vi "NACA_0015_Pressure_with_profile.vi"(3 "Mode":T5, 5 "Traverse line In":T1 {"Row Duration (mins)" format="%#.1f"; "Row No" min=0; "Trace Gas Concentration (%)" min=0.0 format="%#.2f"; "Emission Rate (l/min)" format="%#.2f"; "Tunnel Speed" format="%#.2f"; "Start X" format="%#.2f"; "Start Y" format="%#.2f"; "Start Z" format="%#.2f"; "End X" format="%#.2f"; "End Y" format="%#.2f"; "End Z" format="%#.2f"; "Averaging time (min)" min=0.0 format="%#.2f"}) -> (0 "Error Message":string, 1 "Status":T4, 2 "Traverse line Out":T1 {"Row Duration (mins)" format="%#.1f"; "Row No" min=0; "Trace Gas Concentration (%)" min=0.0 format="%#.2f"; "Emission Rate (l/min)" format="%#.2f"; "Tunnel Speed" format="%#.2f"; "Start X" format="%#.2f"; "Start Y" format="%#.2f"; "Start Z" format="%#.2f"; "End X" format="%#.2f"; "End Y" format="%#.2f"; "End Z" format="%#.2f"; "Averaging time (min)" min=0.0 format="%#.2f"})   [LabVIEW 2011]
uses:
  Gen Trav/Traverse_cluster.ctl
  Gen Trav/Spacing.ctl
  Controls/Multi_run_mode.ctl
  Controls/User_Specific_mode.ctl
  Gen Trav/Multi_Run_Status.ctl
  Gen Trav/Trav_mode.ctl
  Controls/Save_Data.ctl
  Controls/Setup.ctl
  <vilib>/Analysis/1siggen.llb/Ramp Pattern by Delta.vi
  <vilib>/Analysis/1siggen.llb/Ramp Pattern by Samples.vi
  Globals/Extra_Commands_Global.vi
  Globals/Meas_global.vi
  <vilib>/Analysis/NI_AALBase.lvlib
panel:
  out "Profile Points":cluster{dbl[], dbl[]}[](graph)
  out "Wake Profile":cluster{dbl[], dbl[]}(graph)
  in  "stop":bool
  out "Pressure":cluster{dbl[], dbl[]}(graph)
  out "Measurement No":i32
  # "X           Y            Z"
  # "Start"
  # "End"
  # "X           Y            Z"
  # "Start"
  # "End"
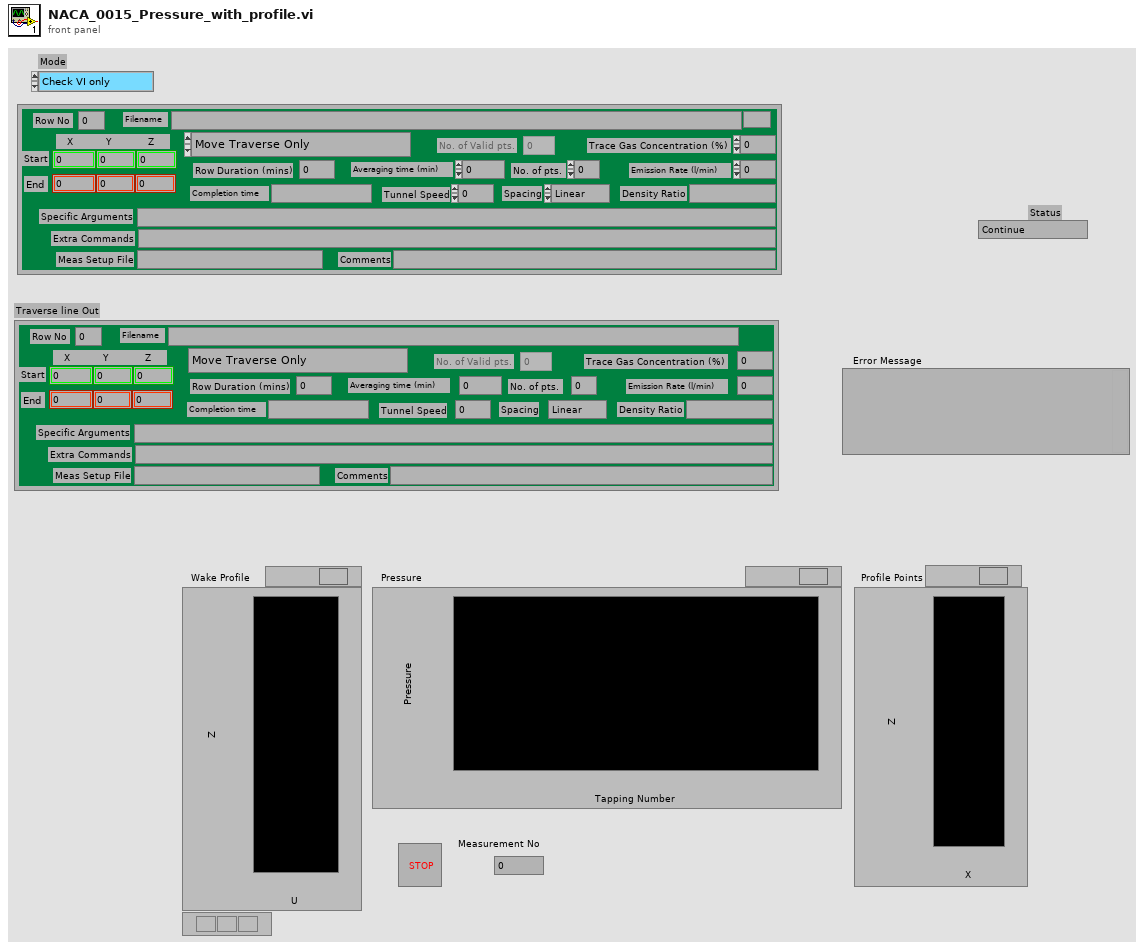
[diagram p1: front panel]
types:
  T1 = typedef "Traverse_cluster.ctl" = cluster{"Start X":dbl, "Start Y":dbl, "Start Z":dbl, "End X":dbl, "End Y":dbl, "End Z":dbl, "No. of pts.":i32, "Spacing":T2, "Filename":path, "Tunnel Speed":dbl, "Averaging time (min)":dbl, "Extra Commands":string, "Specific Arguments":string, "Emission Rate (l/min)":dbl, "Trace Gas Concentration (%)":dbl, "Density Ratio":string, "Comments":string, "Row No":i32, "Row Type Selector":T3, "Completion time":string, "Row Duration (mins)":dbl, "No. of Valid pts.":i32, "Meas Setup File":string}
  T2 = typedef "Spacing.ctl" = enum16{"Linear", "Log", "Gauss", "Specified", "N/A"}
  T3 = typedef "Multi_run_mode.ctl" = enum16{"Move Traverse Only", "Set Tunnel Speed Only", "Set Source Only", "Set Measurement Conditions", "Single Measurement", "Vertical Profile", "Lateral Profile", "Longitudinal Profile", "Explore Volume", "Multi-Axis Profile", "Auto Calibrate", "Meas Fast FID Bkgnd", "Check Beam Power", "Scanning Valve Measurement", "Run VI Named:", "Set ADAM Ch", "Wait (minutes)", "Send Message", "Synchronize With:", "Fall Back to this Row", "Turn Off Row Repeating", "Blank Row", "Traverse 3D Volume"}
  T4 = typedef "Multi_Run_Status.ctl" = enum16{"Continue", "Jump to Next Point", "Jump to Next Row", "Jump To Fall Back", "Terminate Run"}
  T5 = typedef "User_Specific_mode.ctl" = enum16{"Check VI only", "Run VI"}
  T6 = typedef "Trav_mode.ctl" = enum16{"Move traverse", "Read traverse position", "Teach Position"}
  T7 = typedef "Save_Data.ctl" = enum16{"Save No Data", "Save Data"}
  T8 = typedef "Setup.ctl" = enum16{"Run Program", "Show Setup", "Save Current Setup", "Setup Front Panel"}
  T9 = typedef "Status_Cluster.ctl" = cluster{"Status":T4, "Error Type":string, "Error Description":string}
  T10 = typedef "Analysis_info_cluster.ctl" = cluster{"Colour":u32, "Inst type":T11, "Inst name":string, "Symbol":string, "Code name":string, "Extra Info":string, "Inst Array":T12, "Extra Titles":string[], "Extra Values":string[], "U":dbl, "u^2":dbl, "u^3":dbl, "u^4":dbl, "Skew_u":dbl, "Kurt_u":dbl, "Sd Error in Mean":dbl, "% u'/U":dbl, "X":dbl, "Y":dbl, "Z":dbl, "Timescale integral to 25%":dbl, "Sd Error in Variance":dbl, "Calib File":path, "Calib Constants":dbl[], "Output Position":bool, "Full Stats":bool, "Av Sampling Rate":dbl, "Av No of Samples":dbl, "Total Meas Time (s)":dbl, "ADAM Ch Name":string}
  T11 = typedef "Inst_type.ctl" = enum16{"Propeller anemometer", "Raw voltage", "Pressure Transducer", "Pitot-static tube", "Preston tube", "Hot wire", "Cross wire 1", "Cross wire 2", "Generic Linear", "Generic Polynomial", "Generic BackPoly", "Fast FID", "Thermocouple", "Cold wire", "Pulsed Wire", "LDA Vel", "LDA Tran time", "LDA Arr time"}
  T12 = typedef "Instrument_Array.ctl" = enum16{"PWA", "LDA", "Analogue"}
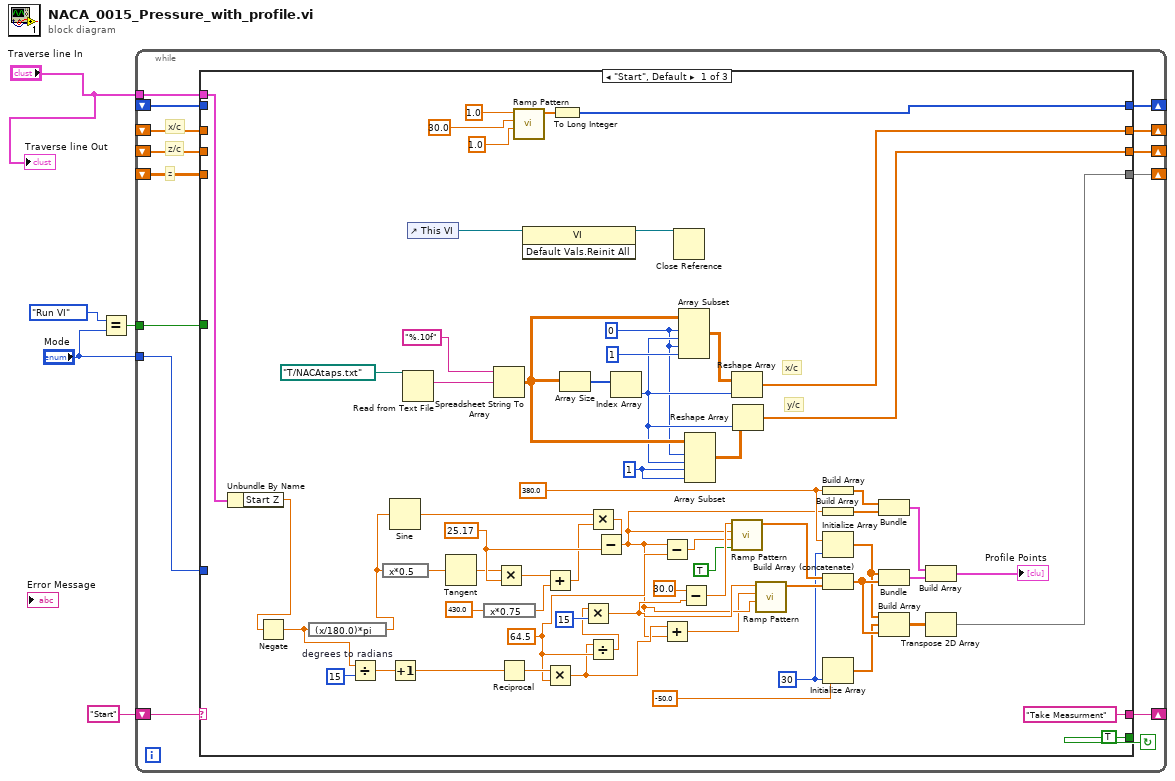
[diagram p0: block diagram]
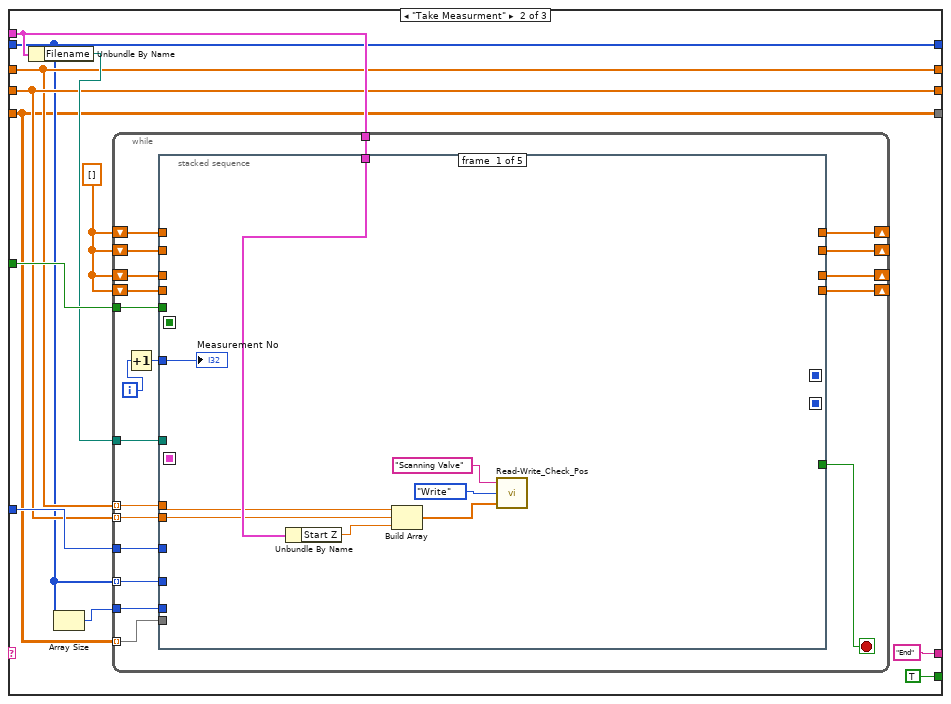
[diagram p2: hidden frame]
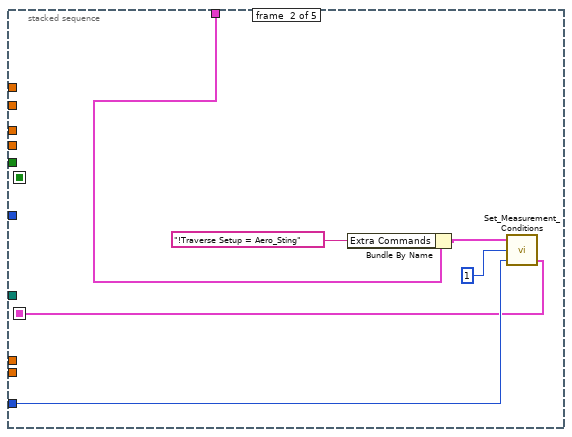
[diagram p3: hidden frame]
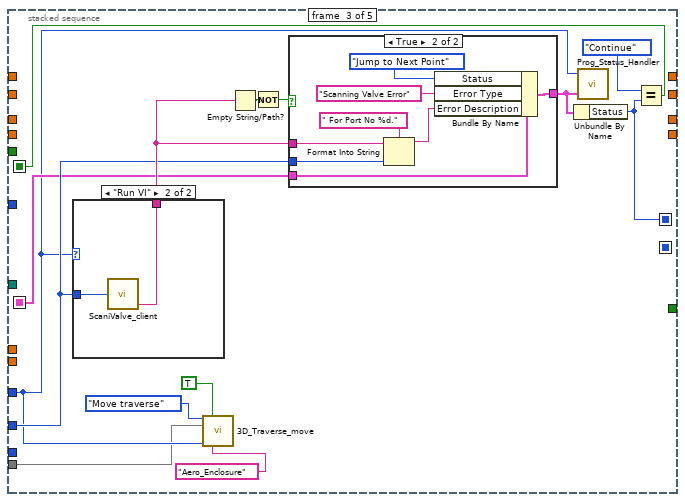
[diagram p4: hidden frame]
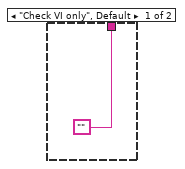
[diagram p5: hidden frame]
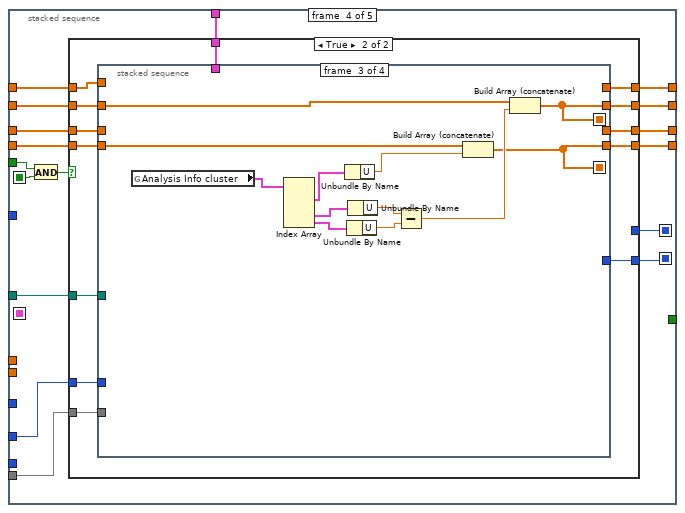
[diagram p7: hidden frame]
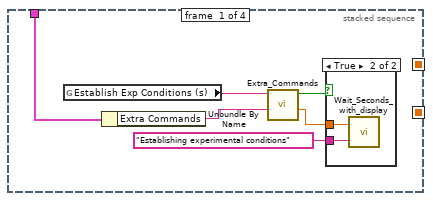
[diagram p9: hidden frame]
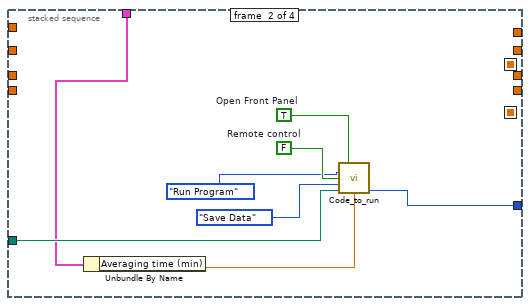
[diagram p11: hidden frame]
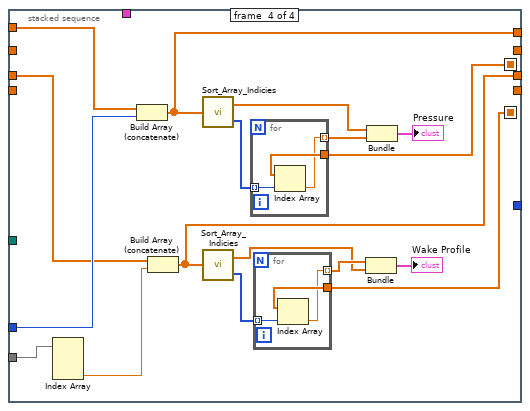
[diagram p12: hidden frame]
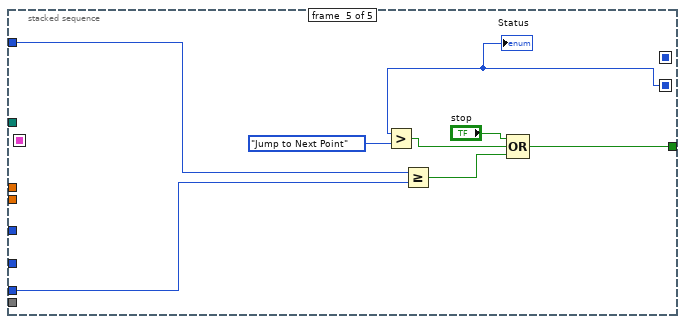
[diagram p13: hidden frame]
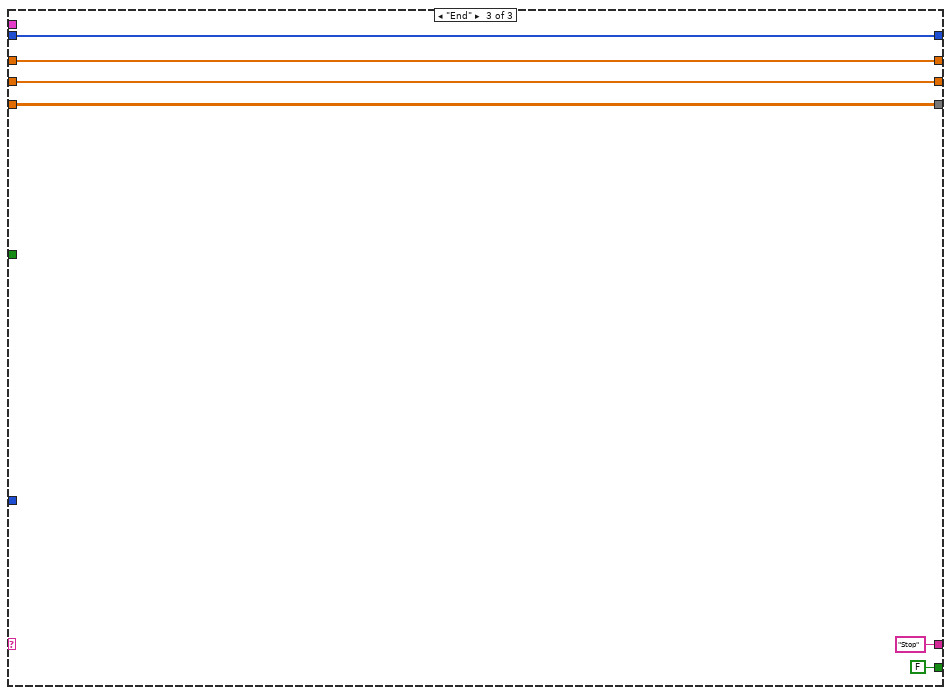
[diagram p14: hidden frame]
diagram:
  n1 = Equal?(x=User_Specific_mode."Run VI" ("Mode"), y="Mode") -> (x = y?=w2:bool)
  n2 = while {
    tunnel: "Traverse line In" -> [w18]
    shift-right: [w17] -> _
    shift-left: "Start" -> [w16]
    tunnel: "Mode" -> [w15]
    tunnel: w2 -> [w14]
    shift-right: [w13] -> _
    shift-left: _ -> [w12]
    shift-right: [w11] -> _
    shift-left: _ -> [w9]
    shift-right: [w10] -> _
    shift-left: _ -> [w8]
    shift-right: [w7] -> _
    shift-left: _ -> [w6]
    stop <- w19 continue-if-true
    # "z"
    # "z/c"
    # "x/c"
    n3 = case shown="\"Start\", Default" w16 {
      tunnel: [TRUE TRUE FALSE] -> w19
      tunnel: w18 -> [w62 w93 _]
      tunnel: ["Take Measurment" "End" "Stop"] -> w17
      tunnel: w15 -> [_ w91 _]
      tunnel: w14 -> [_ w94 _]
      tunnel: [w80 w88 w254] -> w13
      tunnel: w12 -> [_ w88 w254]
      tunnel: [w66 w89 w253] -> w11
      tunnel: [w65 w90 w252] -> w10
      tunnel: w9 -> [_ w89 w253]
      tunnel: w8 -> [_ w90 w252]
      tunnel: [w22 w86 w251] -> w7
      tunnel: w6 -> [_ w86 w251]
      frame "Start", Default {
        w46 = 380.0 ("X")
        w52 = 64.5 ("y")
        w33 = 25.17 ("y")
        w23 = 30 ("dimension size")
        w67 = 1 ("index")
        w68 = 0 ("index")
        # "y/c"
        # "x/c"
        n4 = Unbundle By Name(w62) -> ("Start Z"=w21:dbl)
        n5 = Negate(x=w21) -> (-x=w20:dbl)
        n6 = expression code="(x/180.0)*pi" "degrees to radians"(w20) -> (w43:dbl)
        n7 = Divide(x=w20, y=15) -> (x/y=w54:dbl)
        n8 = expression code="x*0.5"(w43) -> (w26:dbl)
        n9 = Sine(x=w43) -> (sin(x)=w28:dbl)
        n10 = Increment(x=w54) -> (x+1=w55:dbl)
        n11 = Read from Text File(file (use dialog)=path "T:/NACAtaps.txt") -> (text=w76:string)  [unwired: 3 in, 3 out]
        n12 = control-ref of="This VI"() -> (w64:refnum<vi>)
        n13 = Tangent(1:w26) -> (0:w32:dbl)
        n14 = expression code="x*0.75"(430.0) -> (w27:dbl)
        n15 = Spreadsheet String To Array(format string="%.10f", spreadsheet string=w76) -> (array=w72:dbl[][])  [unwired: 2 in]
        n16 = Multiply(x=w32, y=w33) -> (x*y=w31:dbl)
        n17 = Reciprocal(x=w55) -> (1/x=w56:dbl)
        n18 = call-poly <vilib>:"Ramp Pattern.vi"("start"=1.0, "end"=30.0, "delta"=1.0) -> ("Ramp Pattern"=w84:dbl[])  [unwired: 6 in, 2 out]
        n19 = invoke class="VI" method="Default Vals.Reinit All"(reference=w64) -> (reference out=w63:refnum<vi>)  [unwired: 2 in, 2 out]
        n20 = Add(x=w31, y=w27) -> (x+y=w29:dbl)
        n21 = Multiply(x=w56, y=w52) -> (x*y=w51:dbl)
        n22 = To Long Integer(number=w84) -> (32bit integer=w80:i32[])
        n23 = Array Size(array=w72) -> (size(s)=w74:i32[])
        n24 = Multiply(x=w28, y=w29) -> (x*y=w30:dbl)
        n25 = Divide(x=w51, y=w52) -> (x/y=w57:dbl)
        n26 = Multiply(x=w57, y=15 ("dimension size")) -> (x*y=w60:dbl)
        n27 = Subtract(x=w30, y=w33) -> (x-y=w44:dbl)
        n28 = Index Array(array=w74) -> (element=w69:i32)  [unwired: 1 in]
        n29 = Subtract(x=w44, y=w52) -> (x-y=w40:dbl)
        n30 = Add(x=w51, y=w44) -> (x+y=w34:dbl)
        n31 = Close Reference(reference=w63) -> ()  [unwired: 1 in, 1 out]
        n32 = Array Subset(array=w72, index (row)=w68, length (row)=w69, index (col)=w68, length (col)=1 ("length")) -> (w71:dbl[][])
        n33 = Subtract(x=30.0 ("y"), y=w60) -> (x-y=w61:dbl)
        n34 = Array Subset(array=w72, index (row)=w68, length (row)=w69, index (col)=w67, length (col)=w67) -> (w70:dbl[][])
        n35 = Reshape Array(w71, w69) -> (w66:dbl[])
        n36 = call-poly <vilib>:"Ramp Pattern.vi"("exclude end?"=TRUE, "start"=w40, "end"=w44, "samples"=w61) -> ("Ramp Pattern"=w36:dbl[])  [unwired: 6 in, 1 out]
        n37 = Reshape Array(w70, w69) -> (w65:dbl[])
        n38 = call-poly <vilib>:"Ramp Pattern.vi"("start"=w44, "end"=w34, "samples"=w60) -> ("Ramp Pattern"=w37:dbl[])  [unwired: 7 in, 1 out]
        n39 = Build Array(w46) -> (w47:dbl[])
        n40 = Build Array(w44) -> (w45:dbl[])
        n41 = Initialize Array(w46, w23) -> (w41:dbl[])
        n42 = Build Array (concatenate)(w36, w37) -> (w42:dbl[])
        n43 = Initialize Array(-50.0 ("Y"), w23) -> (w38:dbl[])
        n44 = Bundle(w47, w45) -> (w48:cluster{dbl[], dbl[]})  [unwired: 1 in]
        n45 = Bundle(w41, w42) -> (w49:cluster{dbl[], dbl[]})  [unwired: 1 in]
        n46 = Build Array(w41, w38, w42) -> (w39:dbl[][])
        n47 = Build Array(w48, w49) -> (→"Profile Points":cluster{dbl[], dbl[]}[])
        n48 = Transpose 2D Array(2D array=w39) -> (transposed array=w22:dbl[][])
      }
      frame "Take Measurment" {
        w85 = dbl[] []
        n49 = Unbundle By Name(w93) -> ("Filename"=w92:path)
        n50 = Array Size(array=w88) -> (size(s)=w87:i32)
        n51 = while {
          tunnel: w91 -> [w111]
          tunnel: w94 -> [w108]
          tunnel: w92 -> [w116]
          shift-right: [w114] -> _
          shift-left: w85 -> [w115]
          shift-right: [w112] -> _
          shift-left: w85 -> [w113]
          tunnel: w93 -> [w110]
          tunnel: w88 -> [w105] mode=indexing
          tunnel: w89 -> [w104] mode=indexing
          tunnel: w90 -> [w103] mode=indexing
          tunnel: w87 -> [w102]
          tunnel: w86 -> [w101] mode=indexing
          shift-right: [w100] -> _
          shift-left: w85 -> [w99]
          shift-right: [w97] -> _
          shift-left: w85 -> [w98]
          i -> [w107]
          stop <- w109 stop-if-true
          n52 = Increment(x=w107) -> (x+1=w106:i32)
          n53 = stacked-sequence {
            seq-local: [_ _ w139 _ _] -> [_ _ _ w165 _]
            seq-local: [_ _ w138 _ _] -> [_ _ _ w166 _]
            seq-local: [_ _ _ w167 _] -> [_ _ _ _ w244]
            seq-local: [_ w125 _ _ _] -> [_ _ w136 _ _]
            tunnel: w116 -> [_ _ _ w173 _]
            tunnel: w115 -> [_ _ _ w172 _]
            tunnel: [_ _ _ w171 _] -> w114
            tunnel: w113 -> [_ _ _ w170 _]
            tunnel: [_ _ _ w169 _] -> w112
            tunnel: w111 -> [_ w126 w134 _ _]
            tunnel: w110 -> [w123 w127 _ w168 _]
            tunnel: w106 -> [w124 _ _ _ w247]
            tunnel: [_ _ _ _ w245] -> w109
            tunnel: w108 -> [_ _ _ w164 _]
            tunnel: w105 -> [_ _ w137 w162 _]
            tunnel: w104 -> [w122 _ _ _ _]
            tunnel: w103 -> [w121 _ _ _ _]
            tunnel: w102 -> [_ _ _ _ w243]
            tunnel: w101 -> [_ _ w131 w161 _]
            tunnel: [_ _ _ w160 _] -> w100
            tunnel: w99 -> [_ _ _ w159 _]
            tunnel: w98 -> [_ _ _ w158 _]
            tunnel: [_ _ _ w157 _] -> w97
            frame #0 {
              n54 = Unbundle By Name(w123) -> ("Start Z"=w120:dbl)
              n55 = Build Array(w122, w121, w120) -> (w119:dbl[])
              n56 = call "Read-Write_Check_Pos.vi"("Position input"=w119, "Mode"=enum16{"Read", "Write"}."Write", "Traverse Name"="Scanning Valve") -> ()  [unwired: 1 out]
              "Measurement No" <- w124
            }
            frame #1 {
              n57 = Bundle By Name(cluster=w127, "Extra Commands"="!Traverse Setup = Aero_Sting") -> (w130:T1)
              n58 = call "Set_Measurement_Conditions.vi"("Simulate/Run"=w126, "Currently on Point"=1, "Traverse line"=w130) -> ("Status Cluster"=w125:T9)  [unwired: 2 in]
            }
            frame #2 {
              n59 = case shown="\"Run VI\"" w134 {
                tunnel: w137 -> [_ w147]
                tunnel: ["" w146] -> w142
                frame "Check VI only", Default {
                }
                frame "Run VI" {
                  n60 = call "ScaniValve_client.vi"("Port Number"=w147) -> ("Error String"=w146:string)  [unwired: 2 out]
                }
              }
              n61 = call "3D_Traverse_move.vi"("Mode"=Trav_mode."Move traverse", "Route Checking?"=TRUE, "Position"=w131, "Simulate/Run"=w134, "Traverse name"="Aero_Enclosure" ("Traverse Name")) -> ()  [unwired: 8 in, 3 out]
              n62 = Empty String/Path?(string/path=w142) -> (empty?=w144:bool)
              n63 = Not(x=w144) -> (.not. x?=w143:bool)
              n64 = case shown="True" w143 {
                tunnel: w136 -> [w148 w156]
                tunnel: [w148 w153] -> w140
                tunnel: w142 -> [_ w150]
                tunnel: w137 -> [_ w149]
                frame False {
                }
                frame True {
                  n65 = Format Into String(format string=" For Port No %d." ("Format String"), initial string=w150, w149) -> (resulting string=w151:string)  [unwired: 1 in, 1 out]
                  n66 = Bundle By Name(cluster=w156, "Status"=Multi_Run_Status."Jump to Next Point", "Error Type"="Scanning Valve Error" ("t"), "Error Description"=w151) -> (w153:T9)
                }
              }
              n67 = Unbundle By Name(w140) -> ("Status"=w138:T4)
              n68 = call "Prog_Status_Handler.vi"("Status Cluster"=w140, "Simulate/Run"=w134) -> ()  [unwired: 2 out]
              n69 = Equal?(x=Multi_Run_Status."Continue" ("Status"), y=w138) -> (x = y?=w139:bool)
            }
            frame #3 {
              n70 = And(x=w164, y=w165) -> (x .and. y?=w163:bool)
              n71 = case shown="True" w163 {
                tunnel: [w176 w191] -> w167
                tunnel: w173 -> [_ w190]
                tunnel: w172 -> [w178 w189]
                tunnel: [w178 w188] -> w171
                tunnel: w170 -> [w177 w187]
                tunnel: [w177 w186] -> w169
                tunnel: w168 -> [_ w185]
                tunnel: w162 -> [_ w184]
                tunnel: w166 -> [w176 _]
                tunnel: w161 -> [_ w183]
                tunnel: [w174 w182] -> w160
                tunnel: w159 -> [w174 w181]
                tunnel: w158 -> [w175 w180]
                tunnel: [w175 w179] -> w157
                frame False {
                }
                frame True {
                  n72 = stacked-sequence {
                    seq-local: [_ _ w218 _] -> [_ _ _ w231]
                    seq-local: [_ _ w209 _] -> [_ _ _ w226]
                    tunnel: [_ w202 _ _] -> w191
                    tunnel: w190 -> [_ w201 _ _]
                    tunnel: w189 -> [_ _ w219 _]
                    tunnel: [_ _ w218 _] -> w188
                    tunnel: w187 -> [_ _ _ w236]
                    tunnel: [_ _ _ w234] -> w186
                    tunnel: w185 -> [w197 w200 _ _]
                    tunnel: w184 -> [_ _ _ w229]
                    tunnel: w183 -> [_ _ _ w228]
                    tunnel: [_ _ w209 _] -> w182
                    tunnel: w181 -> [_ _ w208 _]
                    tunnel: w180 -> [_ _ _ w221]
                    tunnel: [_ _ _ w220] -> w179
                    frame #0 {
                      n73 = global read "Extra_Commands_Global.vi" "Establish Exp Conditions (s)"() -> (w194:string)
                      n74 = Unbundle By Name(w197) -> ("Extra Commands"=w196:string)
                      n75 = call "Extra_Commands.vi"("String to Search"=w196, "Command"=w194) -> ("Numeric Value"=w195:dbl, "Command Found"=w193:bool)  [unwired: 2 in, 2 out]
                      n76 = case shown="True" w193 {
                        tunnel: w195 -> [_ w199]
                        tunnel: "Establishing experimental conditions" ("Message") -> [_ w198]
                        frame False {
                        }
                        frame True {
                          n77 = call "Wait_Seconds_with_display.vi"("Message"=w198, "Seconds to wait"=w199) -> ()  [unwired: 1 in, 1 out]
                        }
                      }
                    }
                    frame #1 {
                      w205 = TRUE  # Open Front Panel
                      w207 = FALSE  # Remote control
                      n78 = Unbundle By Name(w200) -> ("Averaging time (min)"=w206:dbl)
                      n79 = call "Code_to_run.vi"("Open Front Panel"=w205, "setup"=Setup."Run Program", "Remote control"=w207, "File"=Save_Data."Save Data", "Results Filename"=w201, "Averaging time (min)"=w206) -> ("Status"=w202:T4)  [unwired: 5 in, 4 out]
                    }
                    frame #2 {
                      n80 = global read "Meas_global.vi" "Analysis Info cluster"() -> (w217:T10[])
                      n81 = Index Array(array=w217) -> (element #1=w211:T10, element #3=w212:T10, element #4=w213:T10)  [unwired: 4 in, 1 out]
                      n82 = Unbundle By Name(w211) -> ("U"=w210:dbl)
                      n83 = Unbundle By Name(w213) -> ("U"=w214:dbl)
                      n84 = Unbundle By Name(w212) -> ("U"=w215:dbl)
                      n85 = Subtract(x=w215, y=w214) -> (x-y=w216:dbl)
                      n86 = Build Array (concatenate)(w208, w210) -> (w209:dbl[])
                      n87 = Build Array (concatenate)(w219, w216) -> (w218:dbl[])
                    }
                    frame #3 {
                      n88 = Index Array(array=w228) -> (element #3=w222:dbl)  [unwired: 3 in, 2 out]
                      n89 = Build Array (concatenate)(w236, w229) -> (w234:dbl[])
                      n90 = Build Array (concatenate)(w221, w222) -> (w220:dbl[])
                      n91 = call "Sort_Array_Indicies.vi"("unsorted array"=w234) -> ("sorted array"=w233:dbl[], "Sort Index"=w232:i32[])
                      n92 = call "Sort_Array_Indicies.vi"("unsorted array"=w220) -> ("sorted array"=w223:dbl[], "Sort Index"=w227:i32[])
                      n93 = for {
                        tunnel: w232 -> [w242] mode=indexing
                        tunnel: w231 -> [w241]
                        tunnel: [w240] -> w230 mode=indexing
                        n94 = Index Array(array=w241, index=w242) -> (element=w240:dbl)
                      }
                      n95 = for {
                        tunnel: w227 -> [w239] mode=indexing
                        tunnel: w226 -> [w238]
                        tunnel: [w237] -> w224 mode=indexing
                        n96 = Index Array(array=w238, index=w239) -> (element=w237:dbl)
                      }
                      n97 = Bundle(w224, "sorted array"=w223) -> (→"Wake Profile":cluster{dbl[], "sorted array":dbl[]})  [unwired: 1 out]
                      n98 = Bundle("sorted array"=w233, w230) -> (→"Pressure":cluster{"sorted array":dbl[], dbl[]})  [unwired: 1 out]
                    }
                  }
                }
              }
            }
            frame #4 {
              n99 = Greater?(x=w244, y=Multi_Run_Status."Jump to Next Point" ("Status")) -> (0:w249:bool)
              n100 = Greater Or Equal?(x=w247, y=w243) -> (x >= y?=w248:bool)
              n101 = Compound Arithmetic op=OR("stop", w249, w248) -> (w245:bool)
              "Status" <- w244
            }
          }
        }
      }
      frame "End" {
      }
    }
  }
  "Traverse line Out" <- "Traverse line In"
